vi "LCP Get Max Device Force.vi"(8 "error in (no error)":errorcluster caption="Fehler (Eingang, kein Fehler)", 11 "Pump Handle":i64) -> (0 "error out":errorcluster caption="Fehler (Ausgang)", 3 "Max Force":dbl)   [LabVIEW 2021, in "labbCAN_Pump_API.lvlib"]
doc: "LCP_Func long LCP_CALL LCP_GetFlowIs(dev_hdl hPump, double *pFlowRateIs);"
uses:
  labbCAN_Pump_API.lvlib
  labbCAN_Pump_API.dll
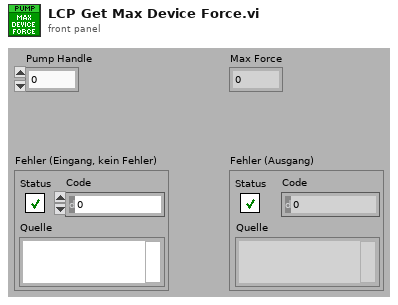
[diagram p1: front panel]
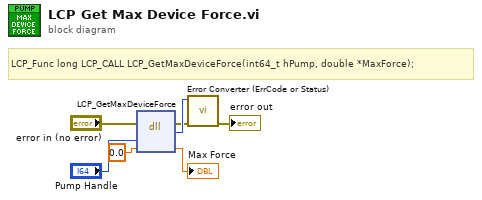
[diagram p0: block diagram]
diagram:
  # "LCP_Func long LCP_CALL LCP_GetMaxDeviceForce(int64_t hPump, double *MaxForce);"
  n1 = dll-call lib="C:/Users/olaja/AppData/Local/CETONI_SDK/labbCAN_Pump_API.*" fn="LCP_GetMaxDeviceForce"(error in="error in (no error)", "hPump"="Pump Handle", "MaxForce"=0.0 ("pFlowRateIs")) -> (error out=w2:errorcluster, "Rückgabetyp"=w3:i32, "MaxForce"=→"Max Force":dbl)  [unwired: 3 in, 1 out]
  n2 = call "Error Converter (ErrCode or Status).vi"("error in (no error)"=w2, "error code"=w3) -> ("error out"=→"error out":errorcluster)  [unwired: 9 in]
